vi "LHF.DB.Mongo.Util.ExtractObjectID.vi"(0 "BsonDocument Refnum in":refnum<k24>, 5 "error in (no error)":errorcluster, 6 "Remove from BSON? (T)":bool=TRUE) -> (14 "BsonDocument Refnum out":refnum<k24>, 15 "_id":string, 19 "error out":errorcluster)   [LabVIEW 2013, in "LHF.DB.Mongo.lvclass"]
uses:
  LHF.DB.Mongo.lvclass
  C:/Users/Ricardo/Desktop/Projetos/LabVIEW-MongoDB/src/Driver/MongoDB.Bson.dll
  LabVIEW-MongoDB/src/Driver/MongoDB.Bson.dll
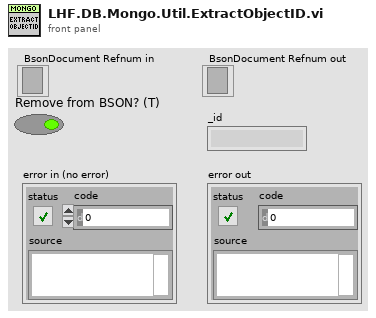
[diagram p1: front panel]
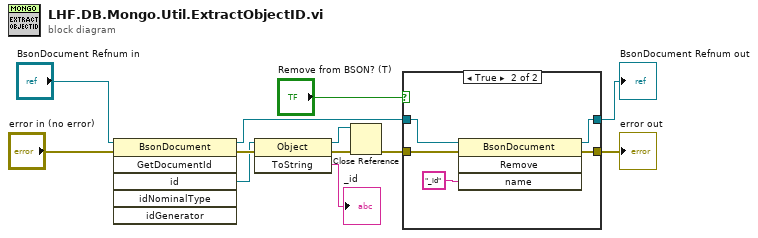
[diagram p0: block diagram]
diagram:
  n1 = invoke class="BsonDocument" method="GetDocumentId"(reference="BsonDocument Refnum in", error in="error in (no error)") -> (reference out=w5:refnum<k24>, error out=w3:errorcluster, "id"=w2:refnum<k24>)  [unwired: 4 in, 3 out]
  n2 = invoke class="Object" method="ToString"(reference=w2, error in=w3) -> (reference out=w11:refnum<k24>, error out=w9:errorcluster, "ToString"=→"_id":string)  [unwired: 1 in]
  n3 = Close Reference(reference=w11, error in (no error)=w9) -> (error out=w10:errorcluster)
  n4 = case shown="True" "Remove from BSON? (T)" {
    tunnel: w10 -> [w13 w18]
    tunnel: [w13 w17] -> w6
    tunnel: w5 -> [w14 w16]
    tunnel: [w14 w15] -> w4
    frame False {
    }
    frame True {
      n5 = invoke class="BsonDocument" method="Remove"(reference=w16, error in=w18, "name"="_id") -> (reference out=w15:refnum<k24>, error out=w17:errorcluster)  [unwired: 1 in, 2 out]
    }
  }
  "error out" <- w6
  "BsonDocument Refnum out" <- w4
